vi "CustomCommandTimer.vi"(9 "numOfSeconds":u32, 10 "startTime":u32, 11 "timeElapsed":u32) -> (3 "stopCommand":bool)   [LabVIEW 2017]
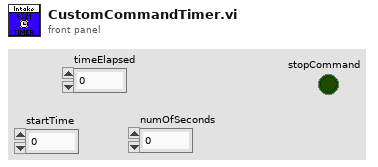
[diagram p1: front panel]
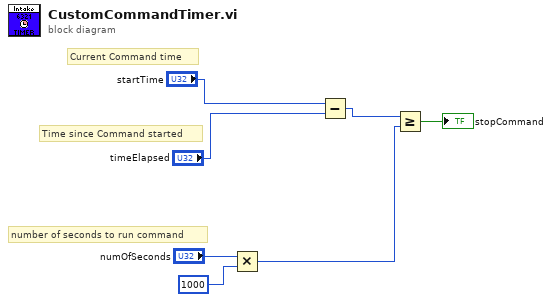
[diagram p0: block diagram]
diagram:
  # "Current Command time"
  # "number of seconds to run command"
  # "Time since Command started"
  n1 = Multiply(x="numOfSeconds", y=u32 1000) -> (x*y=w1:u32)
  n2 = Subtract(x="startTime", y="timeElapsed") -> (x-y=w5:u32)
  n3 = Greater Or Equal?(x=w5, y=w1) -> (x >= y?=→"stopCommand":bool)
